vi "Sampling_Warning_subVI.vi"(8 "error in (no error)":errorcluster) -> (0 "error out":errorcluster)   [LabVIEW 2020]
doc: "Clears warning about sampling."
uses:
  <vilib>/Utility/error.llb/DialogType.ctl
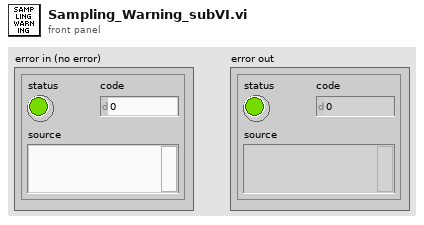
[diagram p1: front panel]
types:
  T1 = typedef "DialogType.ctl" = u16
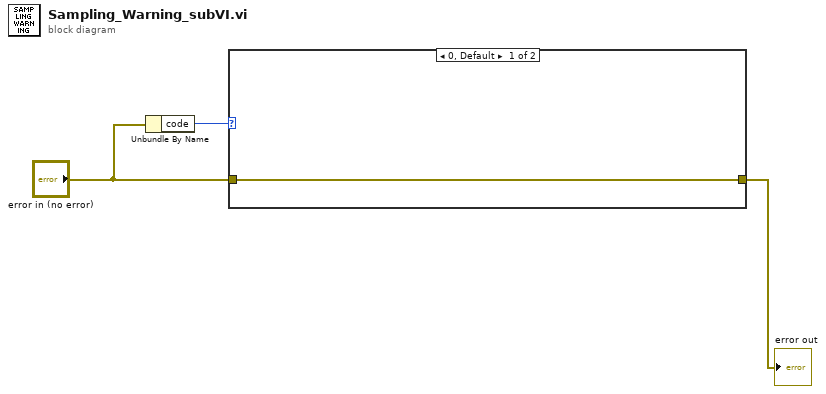
[diagram p0: block diagram]
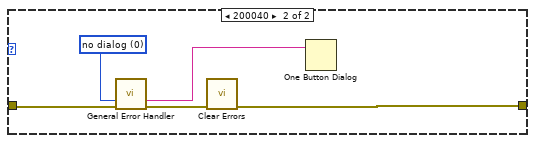
[diagram p2: hidden frame]
diagram:
  n1 = Unbundle By Name("error in (no error)") -> ("code"=w1:i32)
  n2 = case shown="0, Default" w1 {
    tunnel: "error in (no error)" -> [w4 w9]
    tunnel: [w4 w5] -> w3
    frame 0, Default {
    }
    frame 200040 {
      w6 = T1 0 items=["no dialog", "OK message", "continue or stop message", "OK message + warnings", "continue/stop + warnings"] ("type of dialog (OK msg:1)")
      n3 = call <vilib>:"General Error Handler.vi"("type of dialog (OK msg:1)"=w6, "error in (no error)"=w9) -> ("message"=w7:string, "error out"=w8:errorcluster)  [unwired: 9 in, 3 out]
      n4 = call <vilib>:"Clear Errors.vi"("error in (no error)"=w8) -> ("error out"=w5:errorcluster)  [unwired: 5 in, 1 out]
      n5 = One Button Dialog(message=w7) -> ()  [unwired: 1 in, 1 out]
    }
  }
  "error out" <- w3
